vi "List Auto Col Length(Table).vi"(8 "错误输入（无错误）":errorcluster, 10 "Rows":i32=10, 11 "Comm ref":refnum<vi>) -> (0 "错误输出":errorcluster, 3 "引用输出":refnum<vi>)   [LabVIEW 2014]
uses:
  <vilib>/Utility/miscctls.llb/LVRowAndColumnTypeDef.ctl
panel:
  in  "Data":i32[](listbox)
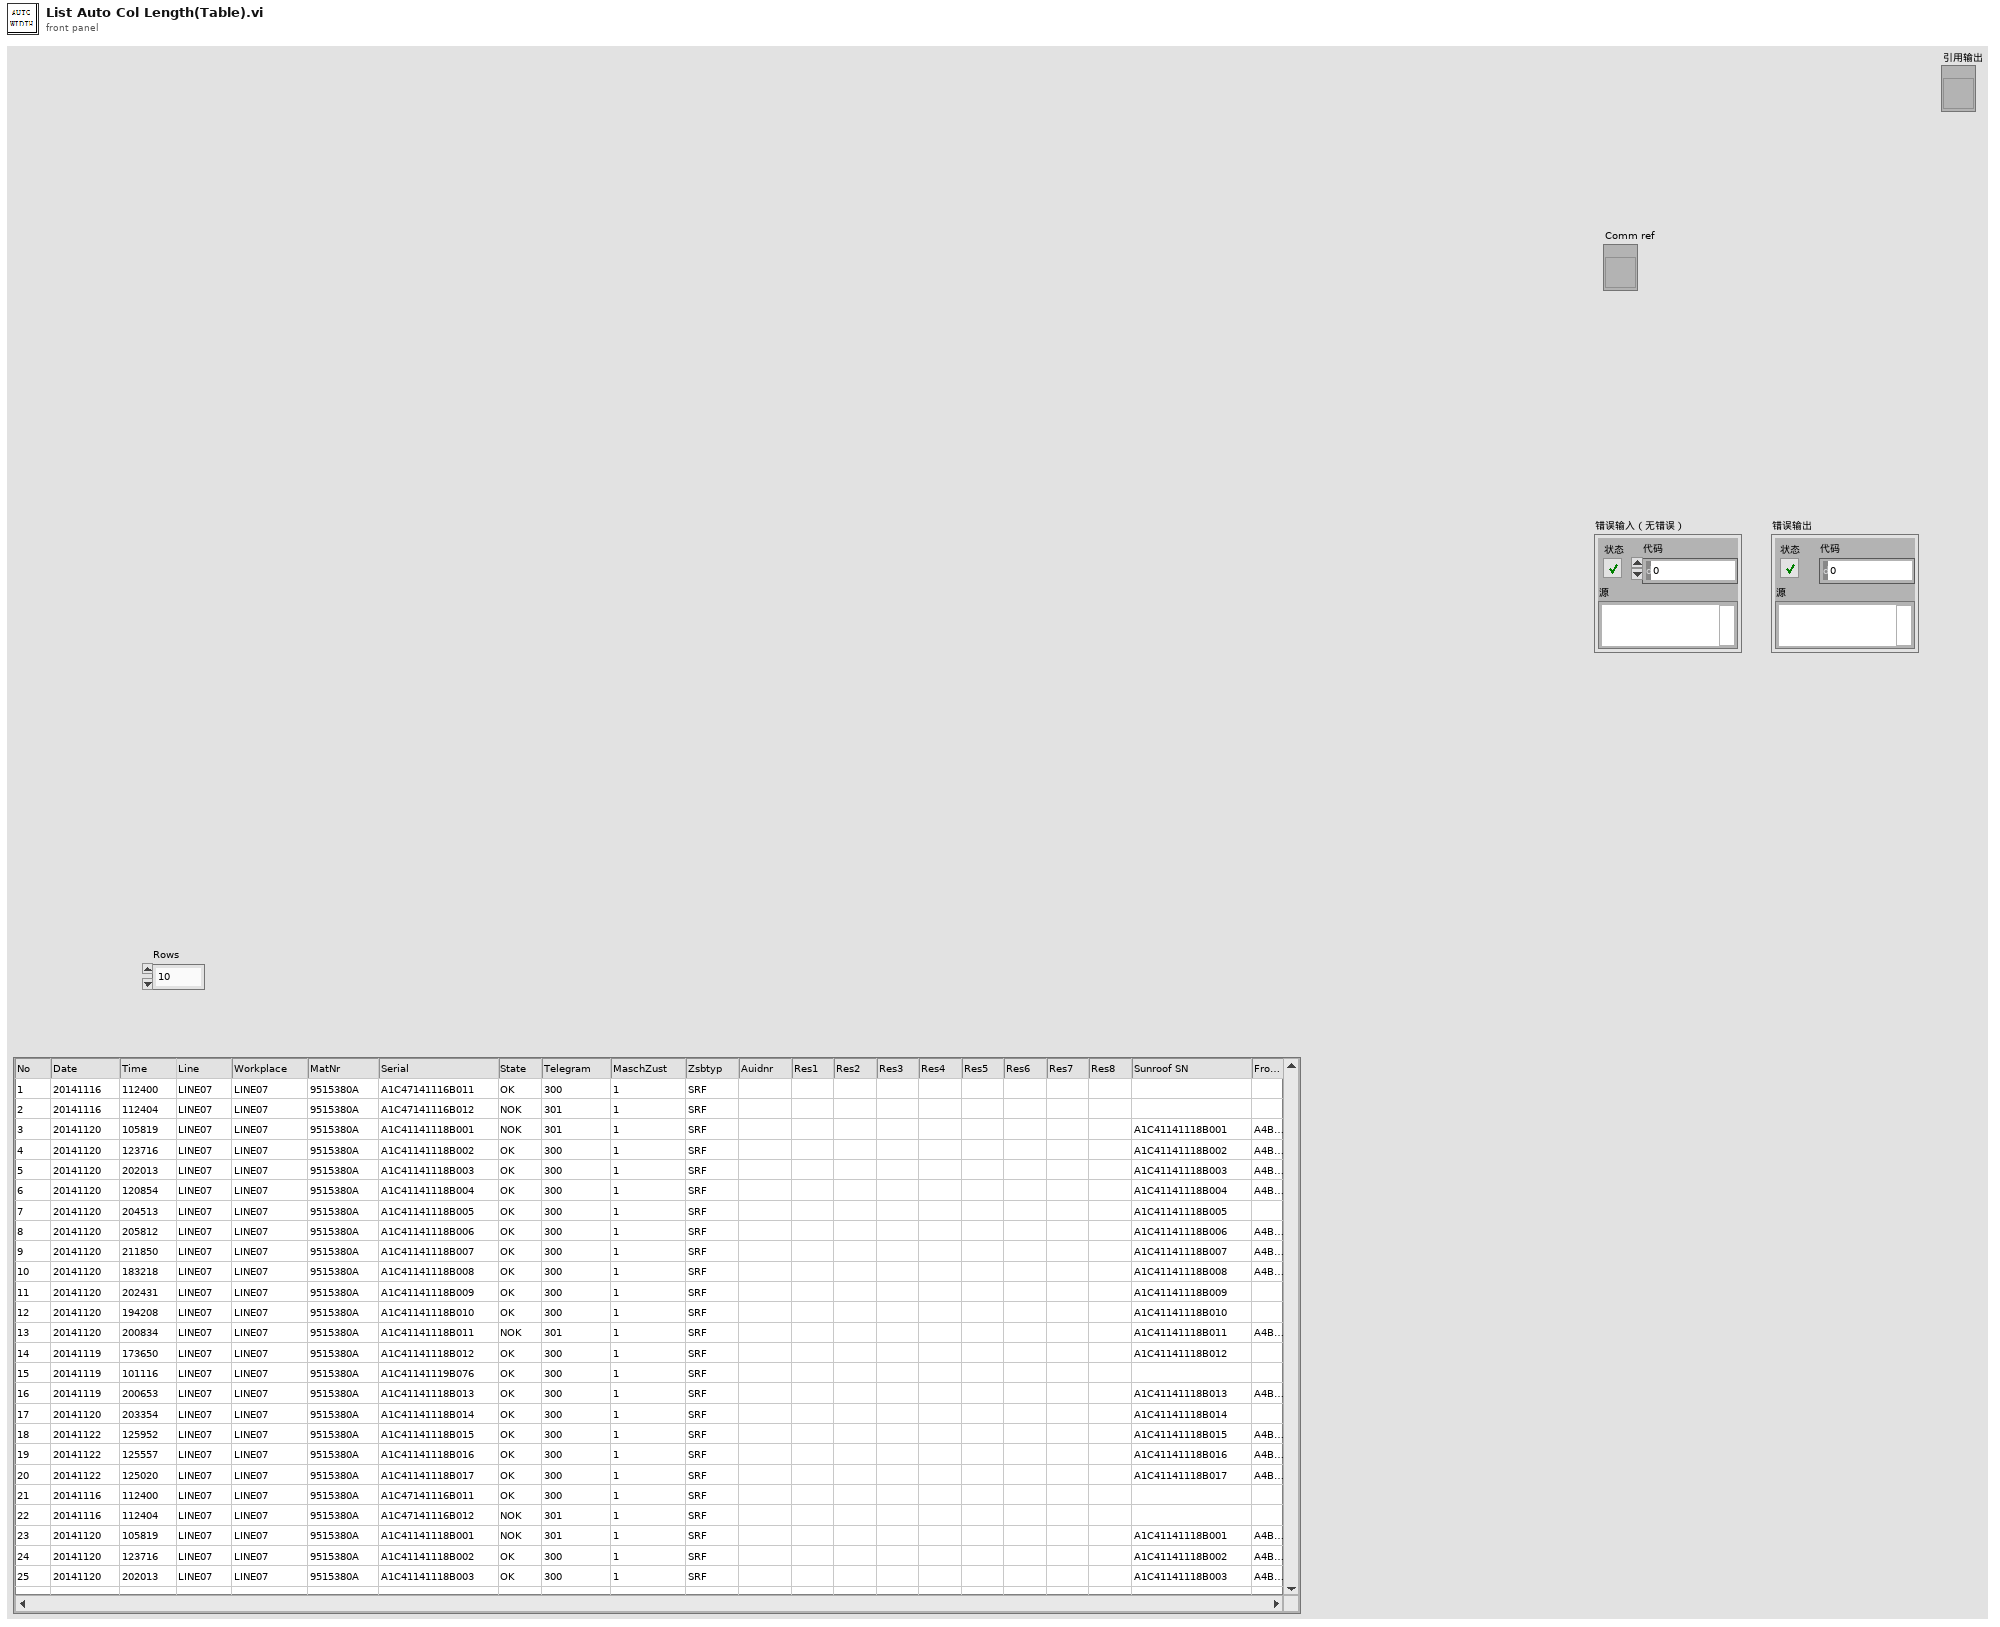
[diagram p1: front panel]
types:
  T1 = typedef "LVRowAndColumnTypeDef.ctl" = cluster{"Row":i32, "Column":i32}
  T2 = typedef "LVFontTypeDef.ctl" = cluster{"Font Name":string, "Size":u16, "Bold":bool, "Italic":bool, "Underline":bool, "Strikeout":bool, "Color":u32}
  T3 = enum16{"User-specified Font", "Application Font", "System Font", "Dialog Font"}
  T4 = cluster{"Font Name:":string, "Size":i16, "Strikeout?":bool, "Italic?":bool, "Underline?":bool, "Outline?":bool, "Shadow?":bool, "Bold?":bool}
  T5 = cluster{"left":i16, "top":i16, "right":i16, "bottom":i16}
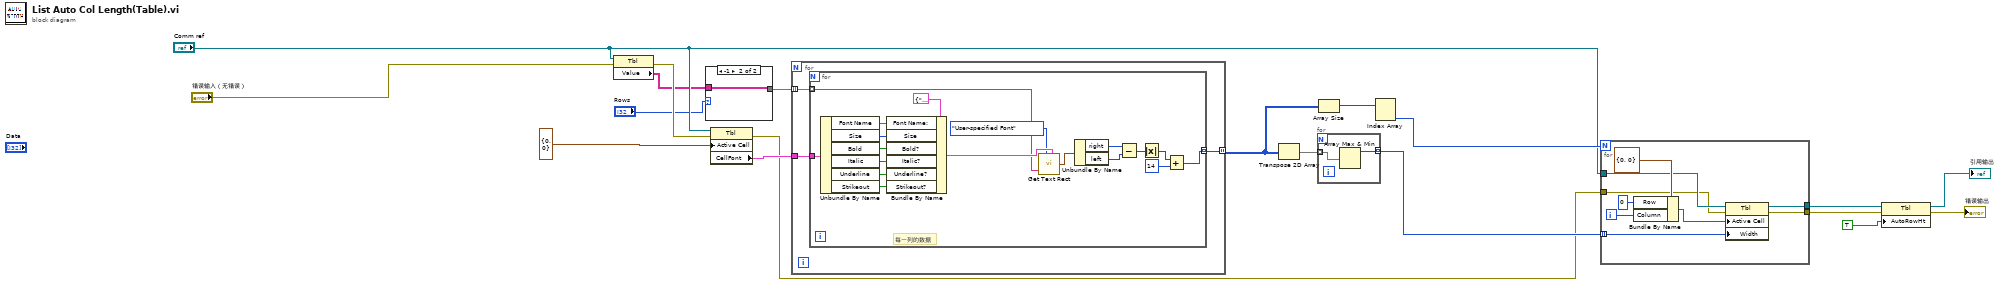
[diagram p0: block diagram]
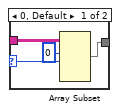
[diagram p2: hidden frame]
diagram:
  n1 = property class="Tbl"(reference="Comm ref", error in="错误输入（无错误）") -> (error out=w11:errorcluster, "Value"=w3:string[][])  [unwired: 1 out]
  n2 = case shown="-1" "Rows" {
    selector: "Rows" -> [w20 _]
    tunnel: w3 -> [w23 w24]
    tunnel: [w22 w24] -> w2
    frame 0, Default {
      n3 = Array Subset(array=w23, index (row)=0 ("索引"), length (row)=w20) -> (w22:string[][])  [unwired: 2 in]
    }
    frame -1 {
    }
  }
  n4 = property class="Tbl"(reference="Comm ref", error in=w11, "Active Cell"=T1 {"Row"=0, "Column"=0} ("Active Cell:Active Cell")) -> (error out=w10:errorcluster, "CellFont"=w18:T2)  [unwired: 1 out]
  n5 = for {
    tunnel: w2 -> [w26] mode=indexing
    tunnel: w18 -> [w27]
    tunnel: [w25] -> w16 mode=indexing
    n6 = for {
      tunnel: w27 -> [w38]
      tunnel: w26 -> [w35] mode=indexing
      tunnel: [w28] -> w25 mode=indexing
      # "每一列的数据"
      n7 = Unbundle By Name(w38) -> ("Font Name"=w44:string, "Size"=w43:u16, "Bold"=w42:bool, "Italic"=w41:bool, "Underline"=w40:bool, "Strikeout"=w39:bool)
      n8 = Bundle By Name(cluster=T4 {"Font Name:"="", "Size"=0, "Strikeout?"=FALSE, "Italic?"=FALSE, "Underline?"=FALSE, "Outline?"=FALSE, "Shadow?"=FALSE, "Bold?"=FALSE} ("[user-specified font]"), "Font Name:"=w44, "Size"=w43, "Bold?"=w42, "Italic?"=w41, "Underline?"=w40, "Strikeout?"=w39) -> (w37:T4)
      n9 = call <vilib>:"Get Text Rect.vi"("desired font(Application)"=T3."User-specified Font", "text"=w35, "[user-specified font]"=w37) -> ("rect"=w34:T5)  [unwired: 6 in]
      n10 = Unbundle By Name(w34) -> ("right"=w33:i16, "left"=w32:i16)
      n11 = Subtract(x=w33, y=w32) -> (x-y=w31:i16)
      n12 = Absolute Value(x=w31) -> (abs(x)=w29:i16)
      n13 = Add(x=w29, y=i16 14) -> (x+y=w28:i16)
    }
  }
  n14 = Transpose 2D Array(2D array=w16) -> (transposed array=w17:i16[][])
  n15 = for {
    tunnel: w17 -> [w47] mode=indexing
    tunnel: [w46] -> w14 mode=indexing
    n16 = Array Max & Min(array=w47) -> (max value=w46:i16)  [unwired: 3 out]
  }
  n17 = Array Size(array=w16) -> (size(s)=w15:i32[])
  n18 = Index Array(array=w15) -> (element #2=w12:i32)  [unwired: 2 in, 1 out]
  n19 = for {
    N: w12 -> [_]
    tunnel: w14 -> [w53] mode=indexing
    tunnel: "Comm ref" -> [w52]
    tunnel: w10 -> [w50]
    tunnel: [w49] -> w9
    tunnel: [w48] -> w8
    i -> [w54]
    n20 = Bundle By Name(cluster=T1 {"Row"=0, "Column"=0} ("Active Cell:Active Cell"), "Row"=0, "Column"=w54) -> (w55:T1)
    n21 = property class="Tbl"(reference=w52, error in=w50, "Active Cell"=w55, "Width"=w53) -> (reference out=w48:refnum<vi>, error out=w49:errorcluster)
  }
  n22 = property class="Tbl"(reference=w8, error in=w9, "AutoRowHt"=TRUE ("Autosizing Row Height")) -> (reference out=→"引用输出":refnum<vi>, error out=→"错误输出":errorcluster)
